vi "abouttest.vi"() -> ()   [LabVIEW 2015]
uses:
  board.vis/Globals.vi
  board.vis/ESLSCDLL.lvlib
panel:
  out "error out":errorcluster
  in  "error in (no error)":errorcluster
  out "boards":u8
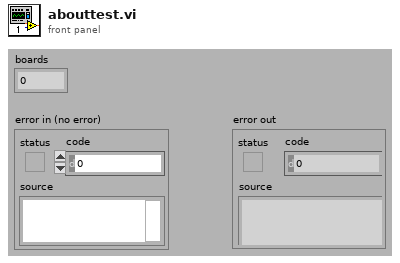
[diagram p1: front panel]
types:
  T1 = enum32{"XCK", "Reg/OutTrig", "VON", "DMA_Act", "ASLS", "STIMER", "BTIMER", "INTRSR", "S1", "S2", "BON", "MEASUREON", "SDAT", "BDAT", "SSHUT", "BSHUT"}
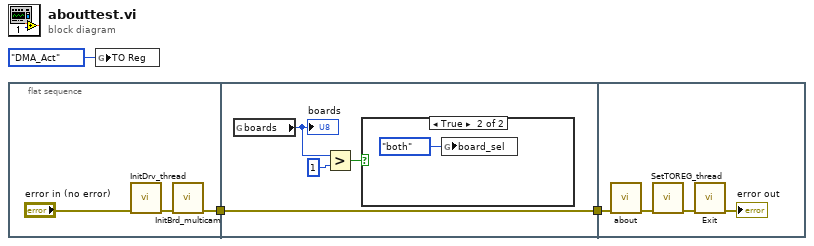
[diagram p0: block diagram]
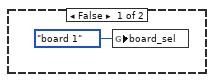
[diagram p2: hidden frame]
diagram:
  n1 = flat-sequence {
    tunnel: [w4] -> w1
    tunnel: [w7] -> w2
    tunnel: w1 -> [w7]
    tunnel: w2 -> [w13]
    frame #0 {
      n2 = call "InitDrv_thread.vi"("error in (no error)"="error in (no error)") -> ("error out"=w6:errorcluster)  [unwired: 10 in]
      n3 = call "InitBrd_multicam.vi"("error in (no error)"=w6) -> ("error out"=w4:errorcluster)  [unwired: 9 in]
    }
    frame #1 {
      n4 = global read "Globals.vi" "boards"() -> (w8:u32)
      "boards" <- w8
      n5 = Greater?(x=w8, y=u32 1) -> (0:w10:bool)
      n6 = case shown="True" w10 {
        frame False {
          n7 = global write "Globals.vi" "board_sel"(enum32{"0", "board 1", "board 2", "both"}."board 1" ("board_sel")) -> ()
        }
        frame True {
          n8 = global write "Globals.vi" "board_sel"(enum32{"0", "board 1", "board 2", "both"}."both" ("board_sel")) -> ()
        }
      }
    }
    frame #2 {
      n9 = call "about.vi"("error in (no error)"=w13) -> ("error out"=w14:errorcluster)  [unwired: 10 in]
      n10 = call "SetTOREG_thread.vi"("error in (no error)"=w14) -> ("error out"=w15:errorcluster)  [unwired: 10 in]
      n11 = call "Exit.vi"("error in (no error)"=w15) -> ("error out"=→"error out":errorcluster)  [unwired: 10 in]
    }
  }
  n12 = global write "Globals.vi" "TO Reg"(T1."DMA_Act" ("TO Reg")) -> ()
